vi "coord_to_str.vi"(10 "y":i32, 11 "x":i32) -> (1 "Column":string, 2 "Row":string, 3 "Combined":string)   [LabVIEW 2015]
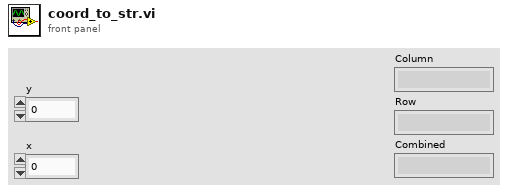
[diagram p1: front panel]
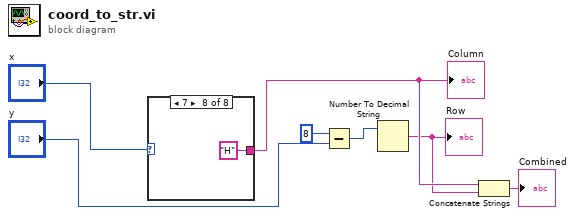
[diagram p0: block diagram]
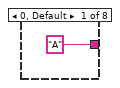
[diagram p2: hidden frame]
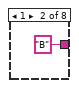
[diagram p3: hidden frame]
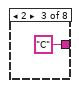
[diagram p4: hidden frame]
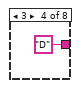
[diagram p5: hidden frame]
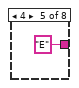
[diagram p6: hidden frame]
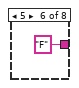
[diagram p7: hidden frame]
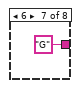
[diagram p8: hidden frame]
diagram:
  n1 = case shown="7" "x" {
    tunnel: ["A" "B" "C" "D" "E" "F" "G" "H"] -> w3
    frame 0, Default {
    }
    frame 1 {
    }
    frame 2 {
    }
    frame 3 {
    }
    frame 4 {
    }
    frame 5 {
    }
    frame 6 {
    }
    frame 7 {
    }
  }
  "Column" <- w3
  n2 = Subtract(x=8, y="y") -> (x-y=w7:i32)
  n3 = Number To Decimal String(number=w7) -> (decimal integer string=w2:string)  [unwired: 1 in]
  "Row" <- w2
  n4 = Concatenate Strings(w3, w2) -> (→"Combined":string)
